vi "Get Waveform Parameters By Name.vi"(0 "RFSG handle":refnum<k15>, 5 "Waveform Name":string, 11 "error in (no error)":errorcluster) -> (4 "RFSG handle out":refnum<k15>, 6 "Waveform":T1={"Name"="Wfm", "Data"=refnum, "Signal Bandwidth (Hz)"=0.0, "PAPR (dB)"=0.0, "Burst Length (s)"=0.0, "Sample Rate"=0.0, "Burst Start Locations"=[], "Burst Stop Locations"=[], "Idle Duration Present?"=FALSE, "Runtime Scaling"=0.0, "Script"=""} {"Runtime Scaling" format="%#_6p"; "Sample Rate" format="%#_6p"; "Burst Length (s)" format="%#_6p"; "PAPR (dB)" format="%.2f"; "Signal Bandwidth (Hz)" format="%#_6p"}, 15 "error out":errorcluster)   [LabVIEW 2019, in "SG.lvlib"]
doc: "Retrieves waveform parameters from the NIRfsgPlayback waveform database based on the waveform name. NOTE - this does not return any value for <b>Waveform.Data</b>. This data cannot be retrieved from the database."
uses:
  SG.lvlib
  Common/Waveform.ctl
  Common/Common.lvlib
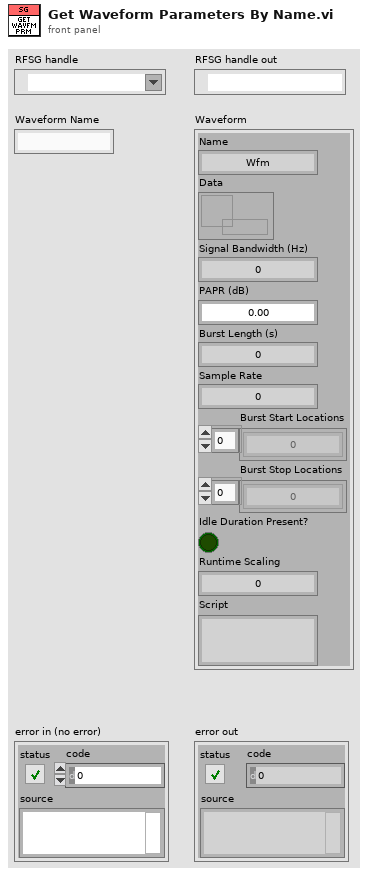
[diagram p1: front panel]
types:
  T1 = typedef "Common.lvlib/Waveform.ctl" = cluster{"Name":string, "Data":refnum<data-value>, "Signal Bandwidth (Hz)":dbl, "PAPR (dB)":dbl, "Burst Length (s)":dbl, "Sample Rate":dbl, "Burst Start Locations":i32[], "Burst Stop Locations":i32[], "Idle Duration Present?":bool, "Runtime Scaling":dbl, "Script":string}
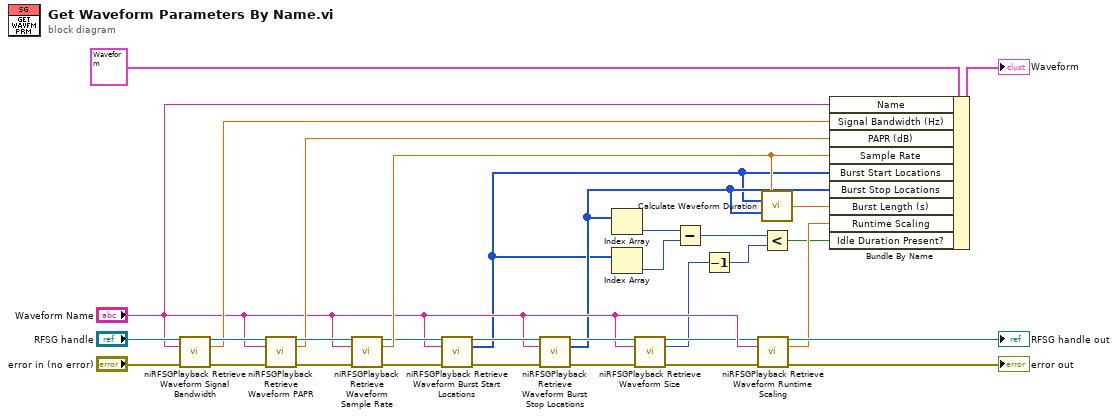
[diagram p0: block diagram]
diagram:
  n1 = call <instrlib>:"niRFSGPlayback Retrieve Waveform Signal Bandwidth.vi"("instrument handle in"="RFSG handle", "waveform name"="Waveform Name", "error in"="error in (no error)") -> ("instrument handle out"=w29:refnum<k15>, "signal bandwidth"=w19:dbl, "error out"=w25:errorcluster)  [unwired: 10 in]
  n2 = call <instrlib>:"niRFSGPlayback Retrieve Waveform PAPR.vi"("instrument handle in"=w29, "waveform name"="Waveform Name", "error in"=w25) -> ("instrument handle out"=w30:refnum<k15>, "PAPR"=w18:dbl, "error out"=w24:errorcluster)  [unwired: 10 in]
  n3 = call <instrlib>:"niRFSGPlayback Retrieve Waveform Sample Rate.vi"("instrument handle in"=w30, "waveform name"="Waveform Name", "error in"=w24) -> ("instrument handle out"=w28:refnum<k15>, "sample rate"=w32:dbl, "error out"=w23:errorcluster)  [unwired: 10 in]
  n4 = call <instrlib>:"niRFSGPlayback Retrieve Waveform Burst Start Locations.vi"("instrument handle in"=w28, "waveform name"="Waveform Name", "error in"=w23) -> ("instrument handle out"=w27:refnum<k15>, "burst start locations"=w1:i32[], "error out"=w22:errorcluster)  [unwired: 10 in]
  n5 = call <instrlib>:"niRFSGPlayback Retrieve Waveform Burst Stop Locations.vi"("instrument handle in"=w27, "waveform name"="Waveform Name", "error in"=w22) -> ("instrument handle out"=w14:refnum<k15>, "burst stop locations"=w2:i32[], "error out"=w13:errorcluster)  [unwired: 10 in]
  n6 = Index Array(array=w2) -> (element=w8:i32)  [unwired: 1 in]
  n7 = Index Array(array=w1) -> (element=w9:i32)  [unwired: 1 in]
  n8 = call <instrlib>:"niRFSGPlayback Retrieve Waveform Size.vi"("instrument handle in"=w14, "waveform name"="Waveform Name", "error in"=w13) -> ("instrument handle out"=w10:refnum<k15>, "waveform size"=w5:i32, "error out"=w11:errorcluster)  [unwired: 10 in]
  n9 = Subtract(x=w8, y=w9) -> (x-y=w7:i32)
  n10 = Decrement(x=w5) -> (x-1=w4:i32)
  n11 = call <instrlib>:"niRFSGPlayback Retrieve Waveform Runtime Scaling.vi"("instrument handle in"=w10, "waveform name"="Waveform Name", "error in"=w11) -> ("instrument handle out"=→"RFSG handle out":refnum<k15>, "runtime scaling"=w15:dbl, "error out"=→"error out":errorcluster)  [unwired: 10 in]
  n12 = call "Calculate Waveform Duration.vi"("Sample Rate"=w32, "Burst Start Locations"=w1, "Burst Stop Locations"=w2) -> ("Burst Length (s)"=w6:dbl)  [unwired: 12 in]
  n13 = Less?(x=w7, y=w4) -> (x < y?=w3:bool)
  n14 = Bundle By Name(cluster=T1 {"Name"="Wfm", "Data"=refnum, "Signal Bandwidth (Hz)"=0.0, "PAPR (dB)"=0.0, "Burst Length (s)"=0.0, "Sample Rate"=0.0, "Burst Start Locations"=[], "Burst Stop Locations"=[], "Idle Duration Present?"=FALSE, "Runtime Scaling"=0.0, "Script"=""} ("Waveform"), "Name"="Waveform Name", "Signal Bandwidth (Hz)"=w19, "PAPR (dB)"=w18, "Sample Rate"=w32, "Burst Start Locations"=w1, "Burst Stop Locations"=w2, "Burst Length (s)"=w6, "Runtime Scaling"=w15, "Idle Duration Present?"=w3) -> (→"Waveform":T1)
